vi "Set Verbose Linker Errors.vi"(8 "error in (no error)":errorcluster, 10 "Verbose Linker Errors? (true)":bool=TRUE, 11 "NI_AB_API_Build in":refnum<class "NI_AB_API_Build.lvclass">) -> (0 "error out":errorcluster, 3 "NI_AB_API_Build out":refnum<class "NI_AB_API_Build.lvclass">)   [LabVIEW 2020, in "NI_AB_API_Build.lvclass"]
uses:
  <vilib>/AppBuilder/AB_API/Build/NI_AB_API_Build.lvclass
  <vilib>/AppBuilder/AB_API/Build/NI_AB_API_Build.lvclass/NI_AB_API_Build.ctl
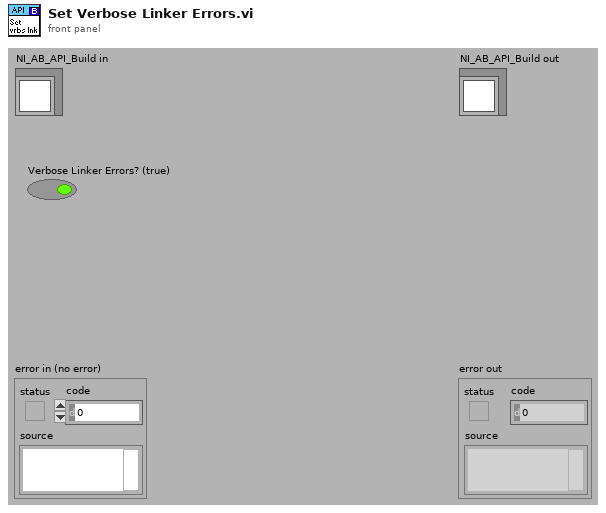
[diagram p1: front panel]
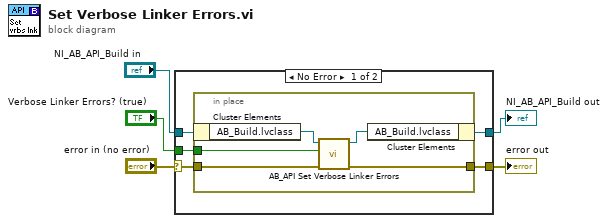
[diagram p0: block diagram]
diagram:
  n1 = case shown="No Error" "error in (no error)" {
    selector: "error in (no error)" -> [w9 w17]
    tunnel: [w8 w17] -> w4
    tunnel: [w6 w16] -> w2
    tunnel: "NI_AB_API_Build in" -> [w7 w16]
    tunnel: "Verbose Linker Errors? (true)" -> [w10 _]
    frame No Error {
      n2 = in-place {
        in-place-border: w10 -> [w15]
        in-place-border: w9 -> [w14]
        in-place-border: [w13] -> w8
        n3 = in-place-cluster #1(w7) -> ("AB_Build.lvclass"=w12:refnum<class "AB_Build.lvclass">)
        n4 = call <vilib>:"AB_API Set Verbose Linker Errors.vi"("error in (no error)"=w14, "Verbose Linker Errors?"=w15, "Build in"=w12) -> ("error out"=w13:errorcluster, "Build out"=w11:refnum<class "AB_Build.lvclass">)  [unwired: 7 in]
        n5 = in-place-cluster #1("AB_Build.lvclass"=w11) -> (w6:refnum<class "NI_AB_API_Build.lvclass">)
      }
    }
    frame Error {
    }
  }
  "error out" <- w4
  "NI_AB_API_Build out" <- w2
